vi "Example Go to Speed.vi"() -> ()   [LabVIEW 2017]
uses:
  <instrlib>/Roboteq Controller KBL1xxx/Roboteq Controller KBL1xxx.lvlib
panel:
  in  "Speed, RPM Slide":dbl(slide) scale=0.0..1000.0
  in  "Stop Button":bool
  out "Sent Command":string
  in  "Controller VISA resource name":refnum<visa-resource-name>
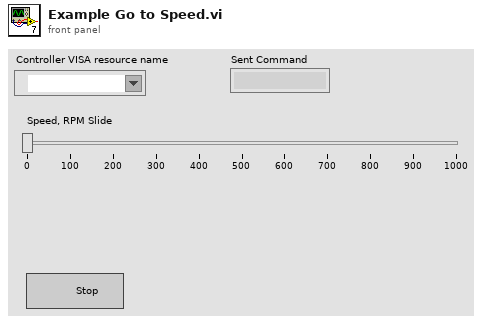
[diagram p1: front panel]
types:
  T1 = typedef "Roboteq Controller KBL1xxx.lvlib/Controller.ctl" = cluster{"VISA resource name out":refnum<visa-resource-name>, "MXRPM":u16}
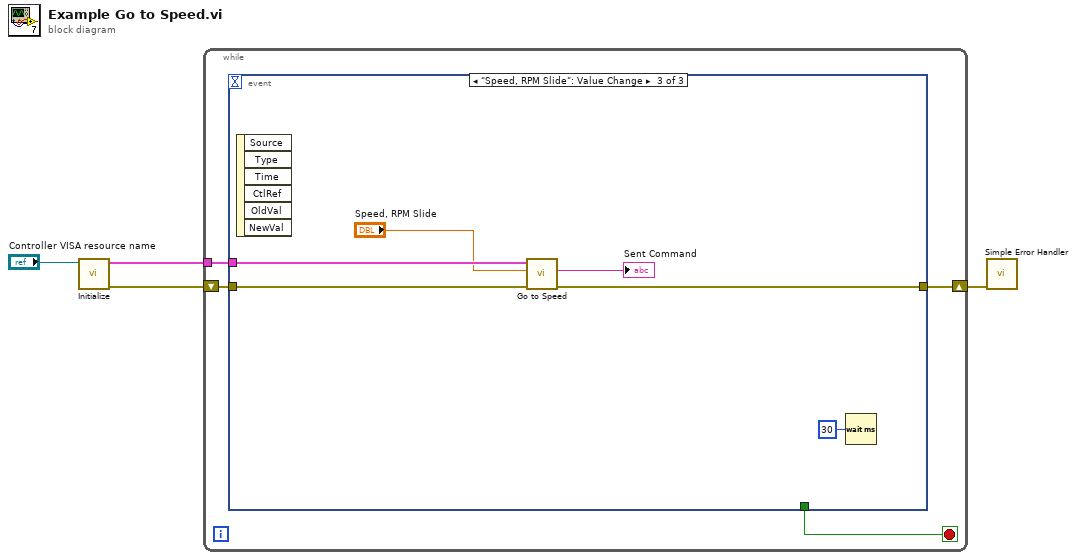
[diagram p0: block diagram]
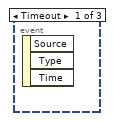
[diagram p2: hidden frame]
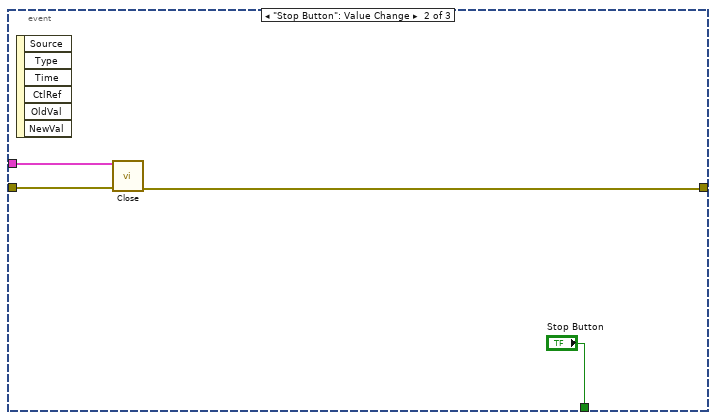
[diagram p3: hidden frame]
diagram:
  n1 = call <instrlib>:"Initialize.vi"("VISA resource name"="Controller VISA resource name") -> ("error out"=w2:errorcluster, "Controller"=w3:T1)  [unwired: 9 in]
  n2 = while {
    tunnel: w3 -> [w7]
    shift-right: [w5] -> w1
    shift-left: w2 -> [w6]
    stop <- w8 stop-if-true
    n3 = event shown="[2] \"Speed, RPM Slide\": Value Change" {
      selector: _ -> [_ _ _]
      dyn-events: _ -> [_ _ _]
      timeout: _ -> [_ _ _]
      tunnel: [_ "Stop Button" _] -> w8
      tunnel: w7 -> [_ w11 w17]
      tunnel: w6 -> [_ w10 w16]
      tunnel: [_ w9 w15] -> w5
      event Timeout {
        n4 = event-data() -> ()  [unwired: 1 in, 3 out]
      }
      event "Stop Button": Value Change {
        n5 = event-data() -> ()  [unwired: 1 in, 6 out]
        n6 = call <instrlib>:"Close.vi"("error in (no error)"=w10, "Controller in"=w11) -> ("error out"=w9:errorcluster)  [unwired: 9 in]
      }
      event "Speed, RPM Slide": Value Change {
        n7 = event-data() -> ()  [unwired: 1 in, 6 out]
        n8 = call <instrlib>:"Go to Speed.vi"("error in (no error)"=w16, "Speed, RPM"="Speed, RPM Slide", "Controller in"=w17) -> ("error out"=w15:errorcluster, "Sent Command"=→"Sent Command":string)  [unwired: 6 in, 1 out]
        n9 = Wait (ms)(milliseconds to wait=u32 30) -> ()  [unwired: 1 out]
      }
    }
  }
  n10 = call <vilib>:"Simple Error Handler.vi"("error in (no error)"=w1) -> ()  [unwired: 4 in, 5 out]
